vi "subSymbolSync.vi"(0 "Data stream":cdb[][](array[numeric]), 9 "Rx Oversample Factor":i32, 11 "error in (no error)":errorcluster) -> (4 "Data stream (out)":cdb[][](array[numeric]), 15 "error out":errorcluster)   [LabVIEW 2011]
uses:
  <vilib>/Analysis/2dsp.llb/Decimate (single shot, CDB).vi
  <vilib>/Analysis/NI_AALPro.lvlib
panel:
  out "antenna index used for sync":i32
  out "powers":dbl[](array[numeric])
  out "max energy sym offset":i32
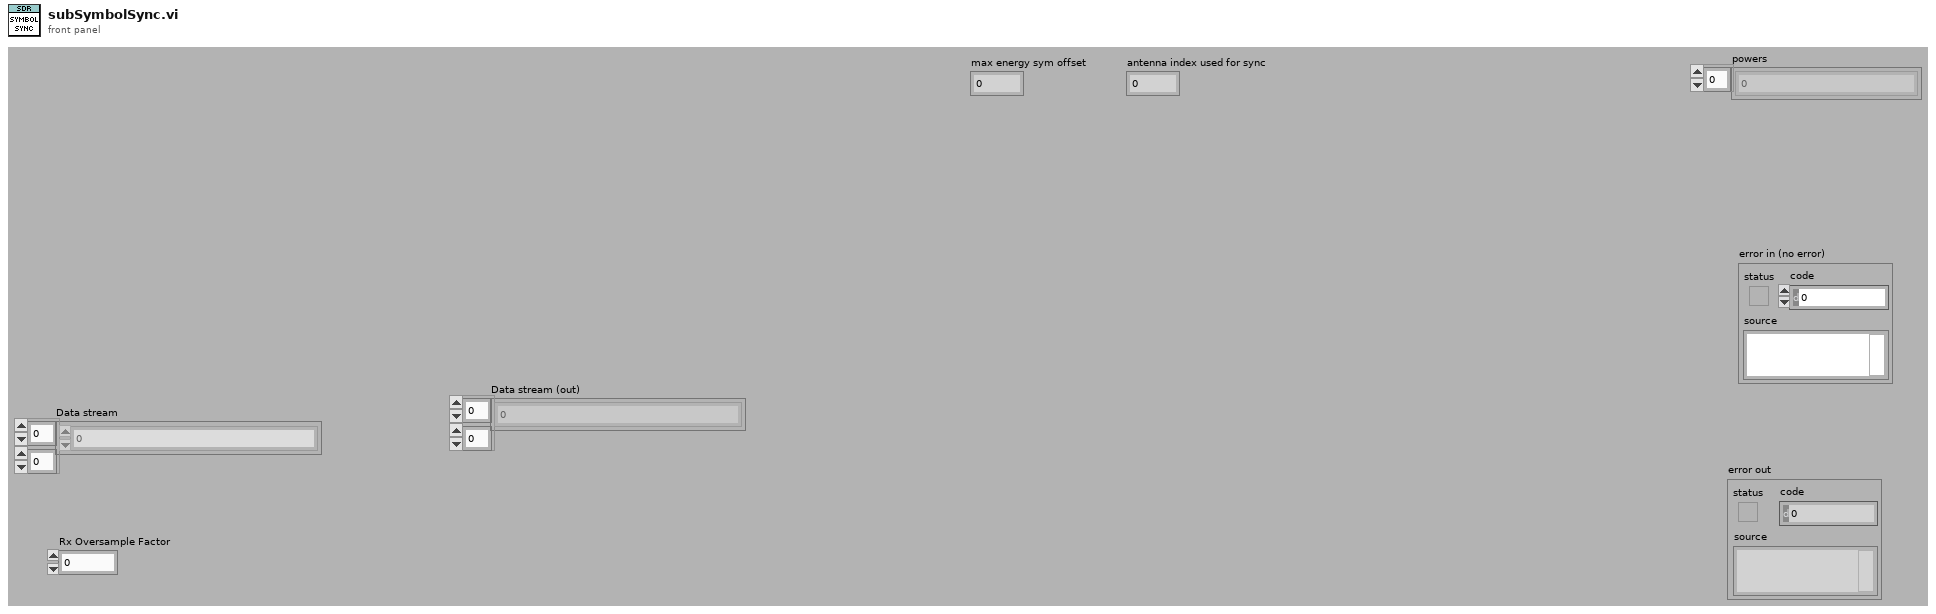
[diagram p1: front panel]
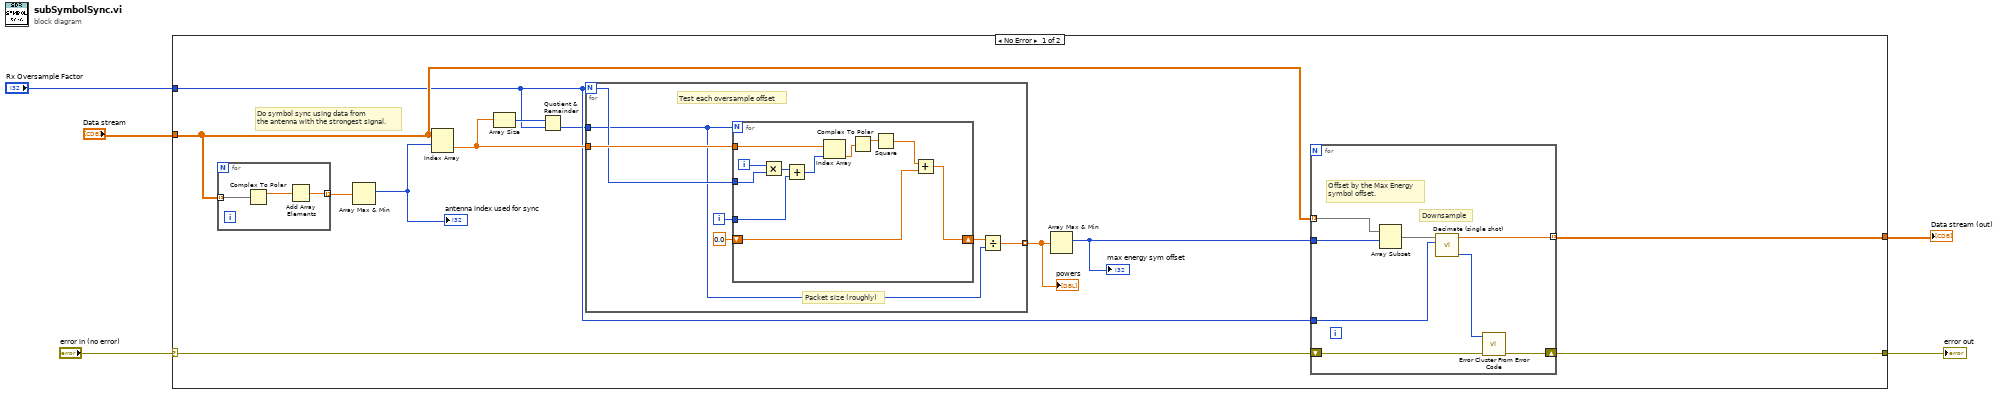
[diagram p0: block diagram]
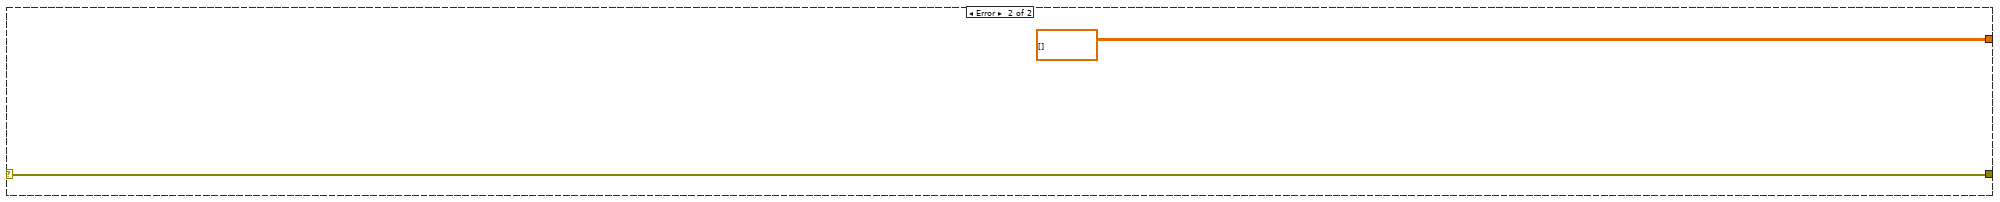
[diagram p2: hidden frame]
diagram:
  n1 = case shown="No Error" "error in (no error)" {
    selector: "error in (no error)" -> [w16 w48]
    tunnel: [w15 w48] -> w4
    tunnel: "Rx Oversample Factor" -> [w7 _]
    tunnel: "Data stream" -> [w11 _]
    tunnel: [w10 cdb[][] []] -> w2
    frame No Error {
      # "Do symbol sync using data from \nthe antenna with the strongest signal."
      n2 = for {
        tunnel: w11 -> [w20] mode=indexing
        tunnel: [w18] -> w13 mode=indexing
        n3 = Complex To Polar(r * e^(i*theta)=w20) -> (r=w19:dbl[])  [unwired: 1 out]
        n4 = Add Array Elements(numeric array=w19) -> (sum=w18:dbl)
      }
      n5 = Array Max & Min(array=w13) -> (max index (indices)=w12:i32)  [unwired: 3 out]
      "antenna index used for sync" <- w12
      n6 = Index Array(array=w11, index (row)=w12) -> (element=w9:cdb[])  [unwired: 1 in]
      n7 = Array Size(array=w9) -> (size(s)=w8:i32)
      n8 = Quotient & Remainder(x=w8, y=w7) -> (floor(x/y)=w6:i32)  [unwired: 1 out]
      n9 = for {
        N: w7 -> [w30]
        tunnel: w9 -> [w31]
        tunnel: [w32] -> w17 mode=indexing
        tunnel: w6 -> [w29]
        i -> [w35]
        # "Packet size (roughly)"
        # "Test each oversample offset"
        n10 = for {
          N: w29 -> [_]
          tunnel: w31 -> [w41]
          tunnel: w30 -> [w45]
          tunnel: w35 -> [w43]
          shift-right: [w36] -> w33
          shift-left: 0.0 -> [w37]
          i -> [w46]
          n11 = Multiply(x=w46, y=w45) -> (x*y=w44:i32)
          n12 = Add(x=w44, y=w43) -> (x+y=w42:i32)
          n13 = Index Array(array=w41, index=w42) -> (element=w40:cdb)
          n14 = Complex To Polar(r * e^(i*theta)=w40) -> (r=w39:dbl)  [unwired: 1 out]
          n15 = Square(x=w39) -> (x^2=w38:dbl)
          n16 = Add(x=w38, y=w37) -> (x+y=w36:dbl)
        }
        n17 = Divide(x=w33, y=w29) -> (x/y=w32:dbl)
      }
      "powers" <- w17
      n18 = Array Max & Min(array=w17) -> (max index (indices)=w14:i32)  [unwired: 3 out]
      "max energy sym offset" <- w14
      n19 = for {
        tunnel: w11 -> [w28] mode=indexing
        tunnel: w7 -> [w26]
        tunnel: [w22] -> w10 mode=indexing
        tunnel: w14 -> [w21]
        shift-right: [w24] -> w15
        shift-left: w16 -> [w25]
        # "Downsample"
        # "Offset by the Max Energy\nsymbol offset."
        n20 = Array Subset(array=w28, index=w21) -> (w27:cdb[])  [unwired: 1 in]
        n21 = call-poly <vilib>:"Decimate (single shot).vi"("decimating factor"=w26, "X"=w27) -> ("error"=w23:i32, "Decimated Array"=w22:cdb[])  [unwired: 1 in, 7 out]
        n22 = call <vilib>:"Error Cluster From Error Code.vi"("error in (no error)"=w25, "error code (0)"=w23) -> ("error out"=w24:errorcluster)  [unwired: 1 in, 6 out]
      }
    }
    frame Error {
    }
  }
  "error out" <- w4
  "Data stream (out)" <- w2
